vi "Import Config UI.vi"() -> (1 "Config":T1, 2 "Cancelled":bool)   [LabVIEW 2020, in "VolatusGUI.lvlib" / "Historian Charting Manager.lvclass"]
uses:
  Historian Charting Manager.lvclass
  JSON Charting Config.ctl
  JSON Chart Group.ctl
  JSON Plot Group.ctl
  JSON Plot Config.ctl
  Import State.ctl
  lv-tree-tools/Tree Map/Tree Map/Extra Entry Info.ctl
  ed8f7000-ce32-49d7-9d48-43a38e53055d.vi
  <vilib>/JDP Science/JSONtext/JSON text to Variant.vi
  <vilib>/JDP Science/JSONtext/LVClass Serializer/JSONtext LVClass Serializer.lvclass
  Historian Charting Manager.lvclass/Historian Charting Manager.ctl
  VolatusGUI.lvlib
  lv-tree-tools/Tree Map/Tree Map/Tree Map.lvclass
panel:
  in  "Cancel":bool
  in  "Accept":bool
  in  "Plot Groups":string(tree)
  in  "Chart Groups":string(tree)
  # "Note: This import will not ensure Plot Groups will be available for selected Chart Groups.\nIf a Plot Group is deselected that is used by a Chart Group, that chart will stay blank."
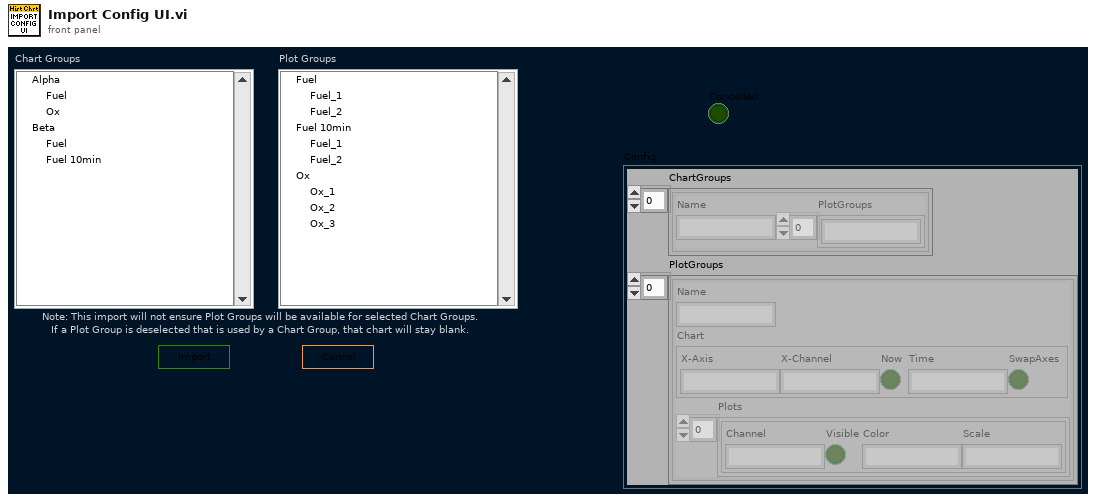
[diagram p1: front panel]
types:
  T1 = typedef "VolatusGUI.lvlib/JSON Charting Config.ctl" = cluster{"ChartGroups":T2[], "PlotGroups":T3[]}
  T2 = typedef "VolatusGUI.lvlib/JSON Chart Group.ctl" = cluster{"Name":string, "PlotGroups":string[]}
  T3 = typedef "VolatusGUI.lvlib/JSON Plot Group.ctl" = cluster{"Name":string, "Chart":cluster{"X-Axis":string, "X-Channel":string, "Now":bool, "Time":string, "SwapAxes":bool}, "Plots":T4[]}
  T4 = typedef "VolatusGUI.lvlib/JSON Plot Config.ctl" = cluster{"Channel":string, "Visible":bool, "Color":string, "Scale":string}
  T5 = typedef "VolatusGUI.lvlib/Historian Charting Manager.lvclass/Import State.ctl" = enum16{"Init", "Browse", "Read", "Select", "Filter"}
  T6 = typedef "Tree Map.lvlib/Tree Map.lvclass/Extra Entry Info.ctl" = cluster{"BG Color":u32, "Symbol":i32}
  T7 = enum32{"Invalid", "Standard", "Closed", "Hidden", "Minimized", "Maximized"}
  T8 = typedef "LVPoint32TypeDef.ctl" = cluster{"Horizontal":i32, "Vertical":i32}
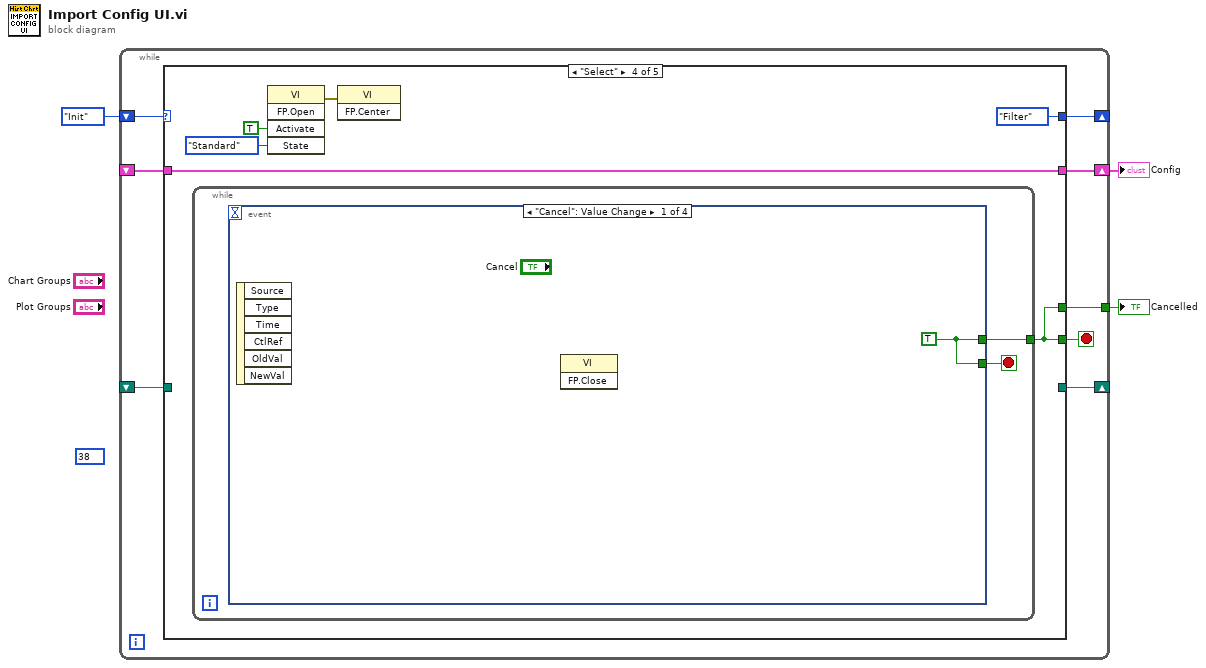
[diagram p0: block diagram]
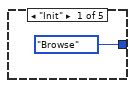
[diagram p2: hidden frame]
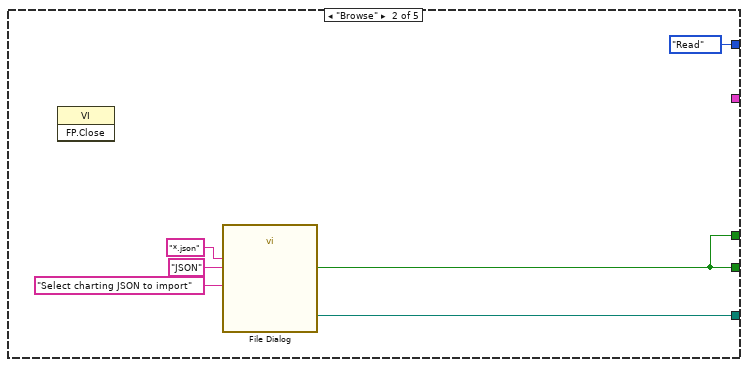
[diagram p3: hidden frame]
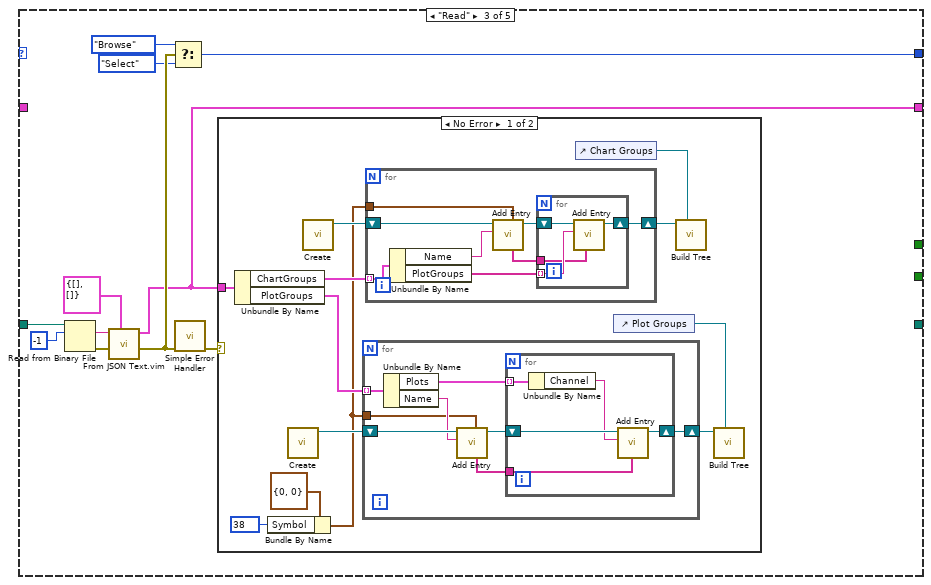
[diagram p4: hidden frame]
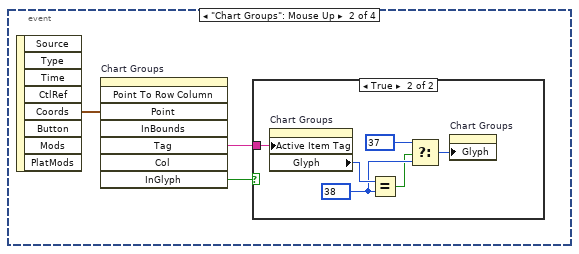
[diagram p6: hidden frame]
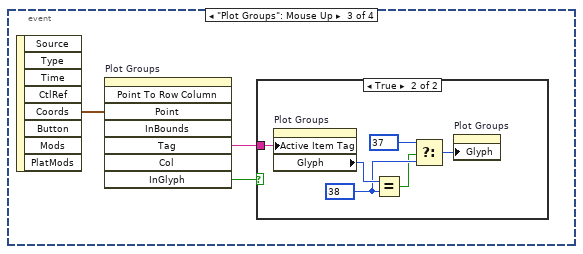
[diagram p8: hidden frame]
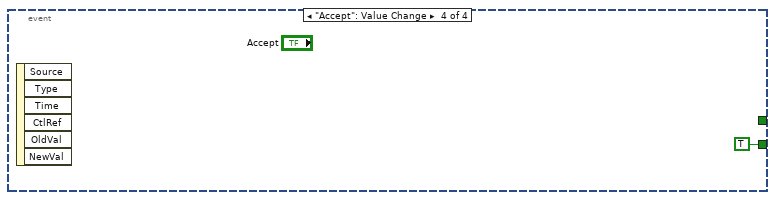
[diagram p10: hidden frame]
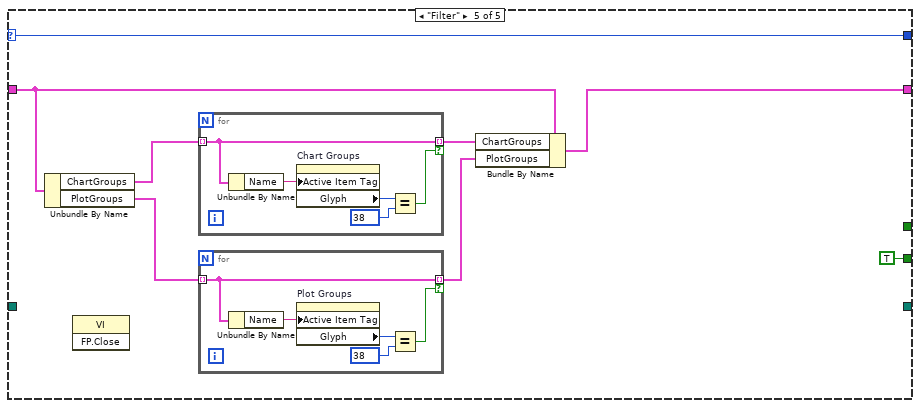
[diagram p11: hidden frame]
diagram:
  (unwired) 38
  n1 = while {
    shift-right: [w10] -> _
    shift-left: Import_State."Init" ("Import State") -> [w11]
    shift-right: [w8] -> _
    shift-left: _ -> [w7]
    shift-right: [w6] -> w1
    shift-left: _ -> [w5]
    tunnel: [w4] -> w2
    stop <- w9 stop-if-true
    n2 = case shown="\"Select\"" w11 {
      selector: w11 -> [_ _ _ _ w102]
      tunnel: [Import_State."Browse" ("Import State") Import_State."Read" ("Import State") w23 Import_State."Filter" ("Import State") w102] -> w10
      tunnel: [_ w13 _ w70 TRUE ("cancelled")] -> w9
      tunnel: [_ w14 _ _ _] -> w8
      tunnel: w7 -> [_ _ w29 _ _]
      tunnel: [_ _ w19 w72 w98] -> w6
      tunnel: w5 -> [_ _ _ w72 w100]
      tunnel: [_ w13 _ w70 _] -> w4
      frame "Init" {
      }
      frame "Browse" {
        n3 = invoke class="VI" method="FP.Close"() -> ()  [unwired: 3 in, 3 out]
        n4 = call "File Dialog"("prompt"="Select charting JSON to import", "pattern (all files)"="*.json", "pattern label"="JSON") -> ("selected path"=w14:path, "cancelled"=w13:bool)  [unwired: 9 in, 2 out]
      }
      frame "Read" {
        n5 = Read from Binary File(10:-1 ("count (1)"), 11:w29) -> (0:w28:errorcluster, 2:w27:string)  [unwired: 4 in, 2 out]
        n6 = call "From JSON Text.vim"("Data Type and Default Value"=T1 {"ChartGroups"=[], "PlotGroups"=[]} ("JSON Charting Config"), "error in (no error)"=w28, "JSON"=w27) -> ("error out"=w24:errorcluster, "Data out"=w19:T1)  [unwired: 7 in]
        n7 = Select(t=Import_State."Browse" ("Import State"), s=w24, f=Import_State."Select" ("Import State")) -> (s? t:f=w23:T5)
        n8 = call <vilib>:"Simple Error Handler.vi"("error in (no error)"=w24) -> ("error out"=w20:errorcluster)  [unwired: 4 in, 4 out]
        n9 = case shown="No Error" w20 {
          tunnel: w19 -> [w41 _]
          frame No Error {
            n10 = Unbundle By Name(w41) -> ("ChartGroups"=w40:T2[], "PlotGroups"=w36:T3[])
            n11 = Bundle By Name(cluster=T6 {"BG Color"=0, "Symbol"=0} ("Extra Info"), "Symbol"=38) -> (w30:T6)
            n12 = call "Create.vi"() -> ("Tree Map out"=w35:refnum<class "Tree Map.lvclass">)  [unwired: 10 in, 1 out]
            n13 = call "Create.vi"() -> ("Tree Map out"=w39:refnum<class "Tree Map.lvclass">)  [unwired: 10 in, 1 out]
            n14 = for {
              tunnel: w36 -> [w49] mode=indexing
              shift-right: [w43] -> w34
              shift-left: w35 -> [w48]
              tunnel: w30 -> [w42]
              n15 = Unbundle By Name(w49) -> ("Plots"=w45:T4[], "Name"=w47:string)
              n16 = call "Add Entry.vi"("Extra Info"=w42, "Name"=w47, "Tree Map in"=w48) -> ("Tree Map out"=w46:refnum<class "Tree Map.lvclass">, "Hierarchy"=w44:string[])  [unwired: 6 in, 1 out]
              n17 = for {
                shift-right: [w50] -> w43
                shift-left: w46 -> [w53]
                tunnel: w45 -> [w54] mode=indexing
                tunnel: w44 -> [w51]
                n18 = Unbundle By Name(w54) -> ("Channel"=w52:string)
                n19 = call "Add Entry.vi"("Parent (None)"=w51, "Name"=w52, "Tree Map in"=w53) -> ("Tree Map out"=w50:refnum<class "Tree Map.lvclass">)  [unwired: 6 in, 2 out]
              }
            }
            n20 = for {
              tunnel: w40 -> [w62] mode=indexing
              shift-right: [w56] -> w38
              shift-left: w39 -> [w61]
              tunnel: w30 -> [w55]
              n21 = Unbundle By Name(w62) -> ("Name"=w60:string, "PlotGroups"=w58:string[])
              n22 = call "Add Entry.vi"("Extra Info"=w55, "Name"=w60, "Tree Map in"=w61) -> ("Tree Map out"=w59:refnum<class "Tree Map.lvclass">, "Hierarchy"=w57:string[])  [unwired: 6 in, 1 out]
              n23 = for {
                shift-right: [w63] -> w56
                shift-left: w59 -> [w66]
                tunnel: w58 -> [w65] mode=indexing
                tunnel: w57 -> [w64]
                n24 = call "Add Entry.vi"("Parent (None)"=w64, "Name"=w65, "Tree Map in"=w66) -> ("Tree Map out"=w63:refnum<class "Tree Map.lvclass">)  [unwired: 6 in, 2 out]
              }
            }
            n25 = control-ref of="Chart Groups"() -> (w37:refnum<vi>)
            n26 = control-ref of="Plot Groups"() -> (w33:refnum<vi>)
            n27 = call "Build Tree.vi"("Tree"=w37, "Tree Map in"=w38) -> ()  [unwired: 8 in, 2 out]
            n28 = call "Build Tree.vi"("Tree"=w33, "Tree Map in"=w34) -> ()  [unwired: 8 in, 2 out]
          }
          frame Error {
          }
        }
      }
      frame "Select" {
        n29 = while {
          tunnel: [w73] -> w70
          stop <- w74 stop-if-true
          n30 = event shown="[0] \"Cancel\": Value Change" {
            selector: _ -> [_ _ _ _]
            dyn-events: _ -> [_ _ _ _]
            timeout: _ -> [_ _ _ _]
            tunnel: [w75 _ _ TRUE] -> w74
            tunnel: [w75 _ _ _] -> w73
            event "Cancel": Value Change {
              w75 = TRUE
              n31 = event-data() -> ()  [unwired: 1 in, 6 out]
              n32 = invoke class="VI" method="FP.Close"() -> ()  [unwired: 3 in, 3 out]
            }
            event "Chart Groups": Mouse Up {
              n33 = event-data() -> ("Coords"=w78:T8)  [unwired: 1 in, 7 out]
              n34 = invoke on="Chart Groups" class="Tree (strict)" method="Point To Row Column"("Point"=w78) -> ("Tag"=w77:string, "InGlyph"=w76:bool)  [unwired: 7 in, 6 out]
              n35 = case shown="True" w76 {
                tunnel: w77 -> [_ w84]
                frame False {
                }
                frame True {
                  w82 = 38
                  n36 = property on="Chart Groups" class="Tree (strict)"("Active Item Tag"=w84) -> ("Glyph"=w83:i32)  [unwired: 2 in, 2 out]
                  n37 = Equal?(x=w83, y=w82) -> (x = y?=w80:bool)
                  n38 = Select(t=37, s=w80, f=w82) -> (s? t:f=w79:i32)
                  n39 = property on="Chart Groups" class="Tree (strict)"("Glyph"=w79) -> ()  [unwired: 2 in, 2 out]
                }
              }
            }
            event "Plot Groups": Mouse Up {
              n40 = event-data() -> ("Coords"=w85:T8)  [unwired: 1 in, 7 out]
              n41 = invoke on="Plot Groups" class="Tree (strict)" method="Point To Row Column"("Point"=w85) -> ("Tag"=w87:string, "InGlyph"=w86:bool)  [unwired: 7 in, 6 out]
              n42 = case shown="True" w86 {
                tunnel: w87 -> [_ w93]
                frame False {
                }
                frame True {
                  w91 = 38
                  n43 = property on="Plot Groups" class="Tree (strict)"("Active Item Tag"=w93) -> ("Glyph"=w92:i32)  [unwired: 2 in, 2 out]
                  n44 = Equal?(x=w92, y=w91) -> (x = y?=w89:bool)
                  n45 = Select(t=37, s=w89, f=w91) -> (s? t:f=w88:i32)
                  n46 = property on="Plot Groups" class="Tree (strict)"("Glyph"=w88) -> ()  [unwired: 2 in, 2 out]
                }
              }
            }
            event "Accept": Value Change {
              n47 = event-data() -> ()  [unwired: 1 in, 6 out]
            }
          }
        }
        n48 = invoke class="VI" method="FP.Open"("Activate"=TRUE ("Activate?"), "State"=T7."Standard") -> (error out=w67:errorcluster)  [unwired: 3 in, 4 out]
        n49 = invoke class="VI" method="FP.Center"(error in=w67) -> ()  [unwired: 2 in, 3 out]
      }
      frame "Filter" {
        n50 = Unbundle By Name(w100) -> ("ChartGroups"=w99:T2[], "PlotGroups"=w96:T3[])
        n51 = invoke class="VI" method="FP.Close"() -> ()  [unwired: 3 in, 3 out]
        n52 = for {
          tunnel: w99 -> [w111] mode=indexing
          tunnel: [w111] -> w97 mode=indexing if=w108
          n53 = Unbundle By Name(w111) -> ("Name"=w112:string)
          n54 = property on="Chart Groups" class="Tree (strict)"("Active Item Tag"=w112) -> ("Glyph"=w110:i32)  [unwired: 2 in, 2 out]
          n55 = Equal?(x=w110, y=38) -> (x = y?=w108:bool)
        }
        n56 = for {
          tunnel: w96 -> [w106] mode=indexing
          tunnel: [w106] -> w95 mode=indexing if=w103
          n57 = Unbundle By Name(w106) -> ("Name"=w107:string)
          n58 = property on="Plot Groups" class="Tree (strict)"("Active Item Tag"=w107) -> ("Glyph"=w105:i32)  [unwired: 2 in, 2 out]
          n59 = Equal?(x=w105, y=38) -> (x = y?=w103:bool)
        }
        n60 = Bundle By Name(cluster=w100, "ChartGroups"=w97, "PlotGroups"=w95) -> (w98:T1)
      }
    }
  }
  "Cancelled" <- w2
  "Config" <- w1
